vi "GetName.vi"(8 "error in (no error)":errorcluster caption="错误输入（无错误）", 11 "TCPServerClass 输入":refnum<class "TCPServerClass.lvclass">) -> (0 "error out":errorcluster caption="错误输出", 2 "IP:Port":string, 3 "TCPServerClass 输出":refnum<class "TCPServerClass.lvclass">)   [LabVIEW 2019, in "TCPServerClass.lvclass"]
uses:
  TCPServerClass.lvclass
  TCPServerClass.lvclass/TCPServerClass.ctl
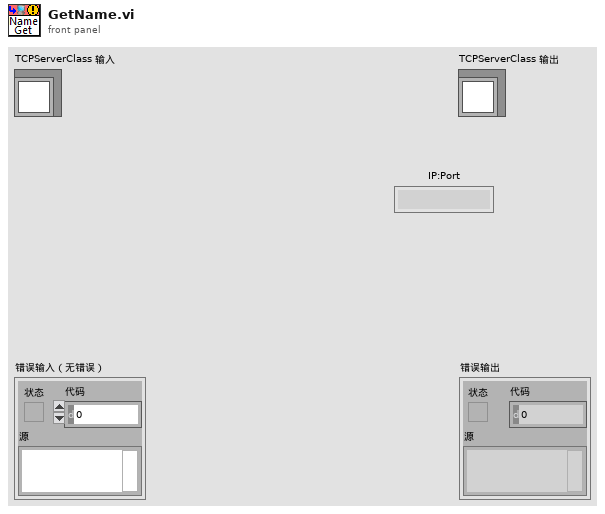
[diagram p1: front panel]
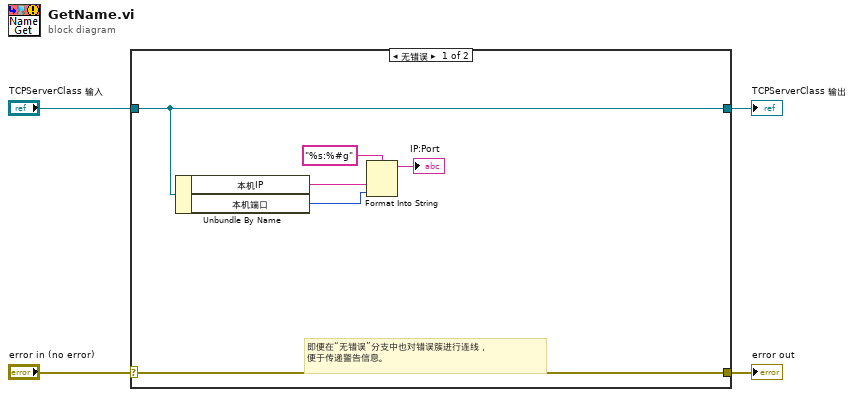
[diagram p0: block diagram]
diagram:
  n1 = case shown="无错误" "error in (no error)" {
    selector: "error in (no error)" -> [w10 w12]
    tunnel: [w10 w12] -> w3
    tunnel: [w9 w11] -> w1
    tunnel: "TCPServerClass 输入" -> [w9 w11]
    frame No Error {
      # "即便在“无错误”分支中也对错误簇进行连线，\n便于传递警告信息。"
      n2 = Unbundle By Name(w9) -> ("本机IP"=w7:string, "本机端口"=w6:u16)
      n3 = Format Into String(format string="%s:%#g" ("格式字符串"), w7, w6) -> (resulting string=→"IP:Port":string)  [unwired: 2 in, 1 out]
    }
    frame Error {
    }
  }
  "error out" <- w3
  "TCPServerClass 输出" <- w1
